vi "getOptStateEstiTestSetting.vi"() -> (3 "Test Setting":T2)   [LabVIEW 2016]
doc: "Get the test setting of OptStateEsti class."
uses:
  StrictDef/InstName.ctl
  OfcFunc.lvlib
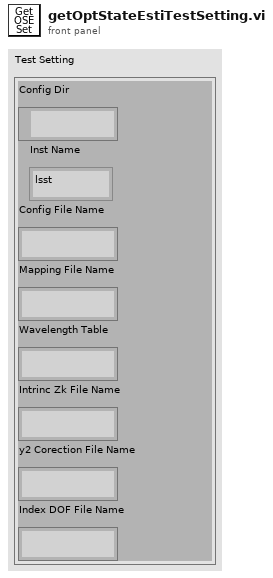
[diagram p1: front panel]
types:
  T1 = typedef "OfcFunc.lvlib/InstName.ctl" = enum16{"lsst", "comcam"}
  T2 = cluster{"Config Dir":path, "Inst Name":T1, "Config File Name":string, "Mapping File Name":string, "Wavelength Table":string, "Intrinc Zk File Name":string, "y2 Corection File Name":string, "Index DOF File Name":string}
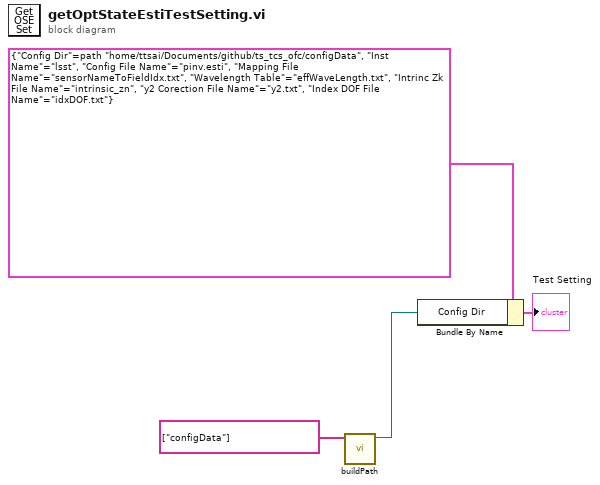
[diagram p0: block diagram]
diagram:
  n1 = call "buildPath.vi"("Path Name List"=string[] ["configData"]) -> ("New Path"=w3:path)  [unwired: 10 in]
  n2 = Bundle By Name(cluster=T2 {"Config Dir"=path "/home/ttsai/Documents/github/ts_tcs_ofc/configData", "Inst Name"=enum."lsst", "Config File Name"="pinv.esti", "Mapping File Name"="sensorNameToFieldIdx.txt", "Wavelength Table"="effWaveLength.txt", "Intrinc Zk File Name"="intrinsic_zn", "y2 Corection File Name"="y2.txt", "Index DOF File Name"="idxDOF.txt"} ("Configuration"), "Config Dir"=w3) -> (→"Test Setting":T2)
